vi "COMBINE HARDWARE defs.vi"(8 "error in":errorcluster) -> (0 "error out":errorcluster, 3 "HARDWARE out":T1={"DRIVE MOTORS"=[], "Controller"=[], "ENCODERS"=[], "GYRO HARDWARE"={"Descr"="GYRO", "Installed?"=FALSE, "SPI Bus"=enum."SPI On-Board, CS0", "AnalogChannel"=enum."AI 0", "Calibrate On Open"=TRUE, "Calibrated Center Voltage"=0.0, "Calibration Time (s)"=2.0, "Sample Rate (Hz)"=100.0, "RefName"="", "stack name"="GYRO"}, "AIR"={"PRESSURE"=[], "COMPRESSOR"={"Descr"="COMPRESSOR", "Installed?"=TRUE, "Pneumatics Control Module"=0, "RefName"="COMPRESSOR", "stack name"="COMPRESSOR"}, "SOLENOIDS"=[]}, "MOTORS"=[], "SERVOS"=[], "SONAR"=[], "RELAY"=[], "LIMIT"=[]} {"MOTORS"."Motor Controller" items=["SPARK", "Existing", "SD540", "TALON SRX", "VICTOR SP", "TALON SR", "JAGUAR", "VICTOR"]; "AIR"."PRESSURE"."warning HIGH" format="%.2f"; "AIR"."PRESSURE"."warning LOW" format="%.2f"; "AIR"."PRESSURE"."nominal value" format="%.2f"; "DRIVE MOTORS"."Motor Controller" items=["SPARK", "Existing", "SD540", "TALON SRX", "VICTOR SP", "TALON SR", "JAGUAR", "VICTOR"]})   [LabVIEW 2017]
uses:
  Controls/def HARDWARE CTRL info.ctl
  Controls/def MOTOR info.ctl
  Controls/ctrl MOTOR CTRLR SELECT.ctl
  <vilib>/Rock Robotics/SystemInterfaces/DIO/FPGA_DIOPWMChannel.ctl
  Controls/def USER CONTROL info.ctl
  <vilib>/Rock Robotics/WPI/Joystick/WPI_JoystickDeviceEnum.ctl
  Controls/def ENCODER info.ctl
  <vilib>/Rock Robotics/SystemInterfaces/DIO/FPGA_DIOChannel.ctl
  <vilib>/Rock Robotics/WPI/Encoder/WPI_EncoderType.ctl
  Controls/def GYRO info.ctl
  <vilib>/Rock Robotics/SystemInterfaces/spilib/spi_bus.ctl
  Controls/ctrl ANALOG CHANNEL SELECT.ctl
  Controls/def AIR PRESSURE info.ctl
  <vilib>/Rock Robotics/SystemInterfaces/AI/FPGA_AIChannel.ctl
  Controls/def COMPRESSOR info.ctl
  Controls/def SOLENOID info.ctl
  <vilib>/Rock Robotics/WPI/Solenoid/WPI_SolenoidChannel.ctl
  <vilib>/Rock Robotics/WPI/Solenoid/WPI_SolenoidValue.ctl
  Controls/def SERVO info.ctl
  Controls/def SONAR info.ctl
  Controls/ctrl SONAR DEVICE SELECT.ctl
  <vilib>/Rock Robotics/WPI/Ultrasonic/WPI_UltrasonicRangeUnits.ctl
  Controls/def RELAY info.ctl
  <vilib>/Rock Robotics/SystemInterfaces/DIO/FPGA_DIORelayChannel.ctl
  <vilib>/Rock Robotics/WPI/Relay/WPI_RelayDirection.ctl
  <vilib>/Rock Robotics/WPI/Relay/WPI_RelayValue.ctl
  Controls/def LIMIT SWITCH info.ctl
  Global  HARDWARE.vi
panel:
  in  "COMBINED HARDWARE cluster in":T1={"DRIVE MOTORS"=[], "Controller"=[], "ENCODERS"=[], "GYRO HARDWARE"={"Descr"="GYRO", "Installed?"=FALSE, "SPI Bus"=enum."SPI On-Board, CS0", "AnalogChannel"=enum."AI 0", "Calibrate On Open"=TRUE, "Calibrated Center Voltage"=0.0, "Calibration Time (s)"=2.0, "Sample Rate (Hz)"=100.0, "RefName"="", "stack name"="GYRO"}, "AIR"={"PRESSURE"=[], "COMPRESSOR"={"Descr"="", "Installed?"=FALSE, "Pneumatics Control Module"=1, "RefName"="", "stack name"=""}, "SOLENOIDS"=[]}, "MOTORS"=[], "SERVOS"=[], "SONAR"=[], "RELAY"=[], "LIMIT"=[]} {"MOTORS"."Motor Controller" items=["SPARK", "Existing", "SD540", "TALON SRX", "VICTOR SP", "TALON SR", "JAGUAR", "VICTOR"]; "AIR"."PRESSURE"."warning HIGH" format="%.2f"; "AIR"."PRESSURE"."warning LOW" format="%.2f"; "AIR"."PRESSURE"."nominal value" format="%.2f"; "DRIVE MOTORS"."Motor Controller" items=["SPARK", "Existing", "SD540", "TALON SRX", "VICTOR SP", "TALON SR", "JAGUAR", "VICTOR"]}
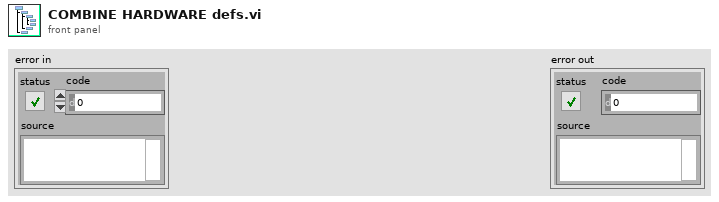
[diagram p1: front panel]
types:
  T1 = typedef "def HARDWARE CTRL info.ctl" = cluster{"DRIVE MOTORS":T2[], "Controller":T5[], "ENCODERS":T7[], "GYRO HARDWARE":T10, "AIR":cluster{"PRESSURE":T13[], "COMPRESSOR":T15, "SOLENOIDS":T16[]}, "MOTORS":T2[], "SERVOS":T19[], "SONAR":T20[], "RELAY":T23[], "LIMIT":T27[]}
  T2 = typedef "def MOTOR info.ctl" = cluster{"Descr":string, "Motor Controller":T3, "PWM ch":T4, "Invert?":bool, "Installed?":bool, "RefName":string, "stack name":string, "remove deadband":bool}
  T3 = typedef "ctrl MOTOR CTRLR SELECT.ctl" = u16
  T4 = typedef "FPGA_DIOPWMChannel.ctl" = enum8{"PWM 0", "PWM 1", "PWM 2", "PWM 3", "PWM 4", "PWM 5", "PWM 6", "PWM 7", "PWM 8", "PWM 9", "PWM MXP 0", "PWM MXP 1", "PWM MXP 2", "PWM MXP 3", "PWM MXP 4", "PWM MXP 5", "PWM MXP 6", "PWM MXP 7", "PWM MXP 8", "PWM MXP 9", "Invalid"}
  T5 = typedef "def USER CONTROL info.ctl" = cluster{"Descr":string, "Installed?":bool, "RefName":string, "JoystickDevice":T6, "Invert Y axis":bool, "Scale":dbl, "AXIS":string, "BUTTONS":string, "POV":string}
  T6 = typedef "WPI_JoystickDeviceEnum.ctl" = enum16{"USB 0", "USB 1", "USB 2", "USB 3", "USB 4", "USB 5"}
  T7 = typedef "def ENCODER info.ctl" = cluster{"Descr":string, "Installed?":bool, "A Channel":T8, "B Channel":T8, "Invert Direction":bool, "Enum":T9, "Gear ratio":dbl, "Cycles per Rev":dbl, "Diameter (in)":dbl[unit], "RefName":string, "stack name":string, "min rate (hz)":dbl, "Samples":u8, "STACK subnames":cluster{"RESET name":string, "STOPPED name":string, "DIRECTION name":string, "RATE name":string, "INSTALLED name":string}}
  T8 = typedef "FPGA_DIOChannel.ctl" = enum8{"DIO 0", "DIO 1", "DIO 2", "DIO 3", "DIO 4", "DIO 5", "DIO 6", "DIO 7", "DIO 8", "DIO 9", "DIO MXP 0", "DIO MXP 1", "DIO MXP 2", "DIO MXP 3", "DIO MXP 4", "DIO MXP 5", "DIO MXP 6", "DIO MXP 7", "DIO MXP 8", "DIO MXP 9", "DIO MXP 10", "DIO MXP 11", "DIO MXP 12", "DIO MXP 13", "DIO MXP 14", "DIO MXP 15", "SPI Port CS1", "SPI Port CS2", "SPI Port CS3", "SPI Port MISO", "SPI Port MOSI", "Invalid"}
  T9 = typedef "WPI_EncoderType.ctl" = enum16{"1x", "2x", "4x"}
  T10 = typedef "def GYRO info.ctl" = cluster{"Descr":string, "Installed?":bool, "SPI Bus":T11, "AnalogChannel":T12, "Calibrate On Open":bool, "Calibrated Center Voltage":dbl, "Calibration Time (s)":dbl, "Sample Rate (Hz)":dbl, "RefName":string, "stack name":string}
  T11 = typedef "spi_bus.ctl" = enum16{"SPI On-Board, CS0", "SPI On-Board, CS1", "SPI On-Board, CS2", "SPI On-Board, CS3", "SPI MXP", "Invalid"}
  T12 = typedef "ctrl ANALOG CHANNEL SELECT.ctl" = enum8{"AI 0", "AI 1", "Invalid"}
  T13 = typedef "def AIR PRESSURE info.ctl" = cluster{"Descr":string, "Installed?":bool, "Channel":T14, "RefName":string, "stack name":string, "MULTIPLIER":dbl, "OFFSET":dbl, "nominal value":dbl, "warning LOW":dbl, "warning HIGH":dbl}
  T14 = typedef "FPGA_AIChannel.ctl" = enum8{"AI 0", "AI 1", "AI 2", "AI 3", "AI MXP 0", "AI MXP 1", "AI MXP 2", "AI MXP 3", "Invalid"}
  T15 = typedef "def COMPRESSOR info.ctl" = cluster{"Descr":string, "Installed?":bool, "Pneumatics Control Module":u8, "RefName":string, "stack name":string}
  T16 = typedef "def SOLENOID info.ctl" = cluster{"Descr":string, "Installed?":bool, "Pneumatics Control Module (0)":u8, "DBL":bool, "SolenoidChannel":T17, "SolenoidChannel":T17, "Default SET":T18, "RefName":string, "Value":string}
  T17 = typedef "WPI_SolenoidChannel.ctl" = enum8{"Solenoid 0", "Solenoid 1", "Solenoid 2", "Solenoid 3", "Solenoid 4", "Solenoid 5", "Solenoid 6", "Solenoid 7", "Invalid"}
  T18 = typedef "WPI_SolenoidValue.ctl" = enum16{"Off", "On", "Forward", "Reverse"}
  T19 = typedef "def SERVO info.ctl" = cluster{"Descr":string, "PWM ch":T4, "Installed?":bool, "Angular range":dbl, "RefName":string, "stack name":string}
  T20 = typedef "def SONAR info.ctl" = cluster{"Descr":string, "Installed?":bool, "Device type":T21, "PING Channel":T8, "ECHO Channel":T8, "RefName":string, "stack name":string, "Samples":i32, "Range Units":T22}
  T21 = typedef "ctrl SONAR DEVICE SELECT.ctl" = enum16{"SRF04 Digital", "MB1010 Digital", "MB1010 Analog", "SRF08 Digital"}
  T22 = typedef "WPI_UltrasonicRangeUnits.ctl" = enum16{"inches", "mm"}
  T23 = typedef "def RELAY info.ctl" = cluster{"Descr":string, "Installed?":bool, "RelayChannel":T24, "Relay Direction":T25, "Relay Value":T26, "RefName":string, "Value":string}
  T24 = typedef "FPGA_DIORelayChannel.ctl" = enum8{"Relay 0", "Relay 1", "Relay 2", "Relay 3", "Invalid"}
  T25 = typedef "WPI_RelayDirection.ctl" = enum16{"Both directions", "Forward only", "Reverse only"}
  T26 = typedef "WPI_RelayValue.ctl" = enum16{"Off", "On", "Forward", "Reverse"}
  T27 = typedef "def LIMIT SWITCH info.ctl" = cluster{"Descr":string, "Installed?":bool, "A Channel":T8, "Normally Closed?":bool, "RefName":string, "stack name":string}
  T28 = cluster{"PRESSURE":T13[], "COMPRESSOR":T15, "SOLENOIDS":T16[]}
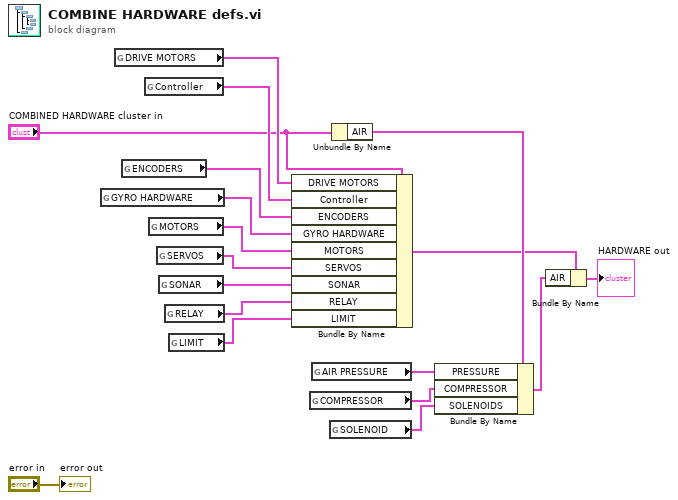
[diagram p0: block diagram]
diagram:
  n1 = global read "Global  HARDWARE.vi" "GYRO HARDWARE"() -> (w14:T10)
  n2 = global read "Global  HARDWARE.vi" "DRIVE MOTORS"() -> (w17:T2[])
  n3 = global read "Global  HARDWARE.vi" "ENCODERS"() -> (w15:T7[])
  n4 = global read "Global  HARDWARE.vi" "Controller"() -> (w16:T5[])
  n5 = global read "Global  HARDWARE.vi" "MOTORS"() -> (w13:T2[])
  n6 = global read "Global  HARDWARE.vi" "SERVOS"() -> (w12:T19[])
  n7 = global read "Global  HARDWARE.vi" "SONAR"() -> (w11:T20[])
  n8 = global read "Global  HARDWARE.vi" "RELAY"() -> (w10:T23[])
  n9 = global read "Global  HARDWARE.vi" "LIMIT"() -> (w9:T27[])
  n10 = Bundle By Name(cluster="COMBINED HARDWARE cluster in", "DRIVE MOTORS"=w17, "Controller"=w16, "ENCODERS"=w15, "GYRO HARDWARE"=w14, "MOTORS"=w13, "SERVOS"=w12, "SONAR"=w11, "RELAY"=w10, "LIMIT"=w9) -> (w3:T1)
  n11 = global read "Global  HARDWARE.vi" "COMPRESSOR"() -> (w5:T15)
  n12 = global read "Global  HARDWARE.vi" "AIR PRESSURE"() -> (w6:T13[])
  n13 = global read "Global  HARDWARE.vi" "SOLENOID"() -> (w4:T16[])
  n14 = Unbundle By Name("COMBINED HARDWARE cluster in") -> ("AIR"=w7:T28)
  n15 = Bundle By Name(cluster=w7, "PRESSURE"=w6, "COMPRESSOR"=w5, "SOLENOIDS"=w4) -> (w2:T28)
  n16 = Bundle By Name(cluster=w3, "AIR"=w2) -> (→"HARDWARE out":T1)
  "error out" <- "error in"
